vi "CheckEncoders.vi"(8 "Target Distance":dbl, 10 "Encoder Left":dbl, 11 "Encoder Right":dbl) -> (2 "Distance Has Been Reached":bool)   [LabVIEW 2016]
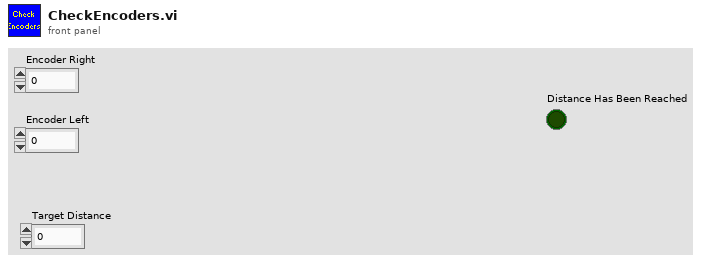
[diagram p1: front panel]
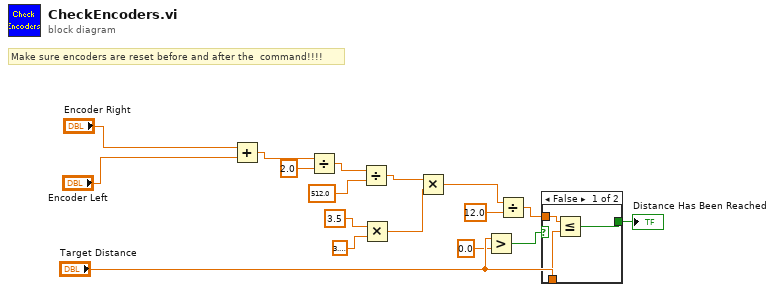
[diagram p0: block diagram]
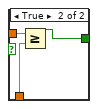
[diagram p2: hidden frame]
diagram:
  # "Make sure encoders are reset before and after the  command!!!!"
  n1 = Add(x="Encoder Right", y="Encoder Left") -> (x+y=w15:dbl)
  n2 = Divide(x=w15, y=2.0) -> (x/y=w13:dbl)
  n3 = Divide(x=w13, y=512.0) -> (x/y=w11:dbl)
  n4 = Multiply(x=3.5 ("y"), y=3.141592653589793) -> (x*y=w9:dbl)
  n5 = Multiply(x=w11, y=w9) -> (x*y=w7:dbl)
  n6 = Greater?(x="Target Distance", y=0.0) -> (0:w3:bool)
  n7 = Divide(x=w7, y=12.0) -> (x/y=w5:dbl)
  n8 = case shown="False" w3 {
    tunnel: w5 -> [w19 w23]
    tunnel: "Target Distance" -> [w20 w22]
    tunnel: [w18 w21] -> w4
    frame False {
      n9 = Less Or Equal?(x=w19, y=w20) -> (x <= y?=w18:bool)
    }
    frame True {
      n10 = Greater Or Equal?(x=w23, y=w22) -> (x >= y?=w21:bool)
    }
  }
  "Distance Has Been Reached" <- w4
